vi "LabVIEW CI Startup VI.vi"   [LabVIEW 2014]
uses:
  Actors/CI Mediator/CI Mediator/CI Mediator.lvclass
  <vilib>/ActorFramework/Actor/Actor.lvclass
panel:
  # "LabVIEW CI Service"
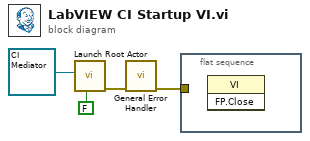
[diagram p0: block diagram]
diagram:
  n1 = call <vilib>:"Launch Root Actor.vi"("Open Actor Core front panel? (F)"=FALSE, "Actor"=refnum<class "CI Mediator.lvclass"> refnum ("CI Mediator.lvlib:CI Mediator.lvclass")) -> ("error out"=w2:errorcluster)  [unwired: 8 in, 1 out]
  n2 = call <vilib>:"General Error Handler.vi"("error in (no error)"=w2) -> ("error out"=w1:errorcluster)  [unwired: 10 in, 4 out]
  n3 = flat-sequence {
    tunnel: w1 -> [_]
    frame #0 {
      n4 = invoke class="VI" method="FP.Close"() -> ()  [unwired: 3 in, 3 out]
    }
  }
